vi "top_loop.vi"(0 "Input parameters":T4={"Measurement type"=enum."Debug", "Sensor type"=enum."HPK_8in_271ch", "Identifier"="test.txt", "Open after execution?"=FALSE, "Plot after execution?"=FALSE, "Display channel"=0, "Voltage Delay (s)"=0.5, "Switch Delay (s)"=0.01, "VISA resource name source"="", "VISA resource name DMM"="", "VISA resource name LCR"="", "Compliance  Level (A)"=10.0, "Voltage Limit (V)"=1000.0, "Data storage location"="", "Scan voltages"="", "Use source as DMM?"=FALSE, "LCR signal frequenzy (Hz)"=10.0, "DMM device"=enum."Keithley2001", "Sampling number"=1, "Use env. sensors on"=enum."Sensirion sht1x/7x", "Switchboard Handle"=0, "Use Switchboard"=FALSE, "LCR signal voltage (V)"=10000.0, "Repeat"=1, "Scan voltages IV"="", "Scan voltages CV"="", "Hex pad numbers?"=FALSE, "Set measurement type"=enum."Debug", "Custom pad scan"="", "IV voltage Delay (s)"=0.5, "CV voltage Delay (s)"=0.5, "Needle measurement?"=FALSE, "Comments"="test.txt", "LCR signal frequenzy (kHz)"=10.0, "Compliance  Level (uA)"=10.0, "Open Correction Array"=array2304x3[6912 elements], "Current set voltage"=0.0, "Last set voltage"=0.0, "Current channel"=0, "Last OpenCorrection index"=-1, "Total curr/vltg every x steps"=10, "Current channel iteration"=0, "No CV corrections"=FALSE, "Mapfile"="", "Corrfile"="", "IV voltage file"=path "", "CV voltage file"=path "", "IV Switch Delay (s)"=0.01, "CV Switch Delay (s)"=0.01, "Invert polarity"=FALSE, "Set debug dirs"=FALSE, "Is n on p"=FALSE, "Source interlock?"=TRUE, "Voltage file used?"=FALSE, "Pad mask"="", "Mask pad above (uA)"=1.0, "LCR device"=enum."LCR_E4980", "Source device"=enum."Source_2410", "HexPlot binary path"="", "PadReductionFactor"=1.0, "Temperature degC"="", "Fluence [neq]"="", "Annealing [min]"=""} {"CV Switch Delay (s)" format="%#_13g"; "IV Switch Delay (s)" format="%#_13g"; "Last set voltage" format="%#_13g"; "Current set voltage" format="%#_13g"; "CV voltage Delay (s)" format="%#_13g"; "IV voltage Delay (s)" format="%#_13g"; "Voltage Limit (V)" format="%#_13g"; "Voltage Delay (s)" format="%#_13g"; "Switch Delay (s)" format="%#_13g"}, 2 "?":refnum<k7>(container), 5 "Dynamic data":T3, 7 "Front_panel_refs":T2, 11 "error in (no error)":errorcluster, 12 "Environmental data":T1) -> (4 "Input parameters out":T4={"Measurement type"=enum."Debug", "Sensor type"=enum."HPK_8in_271ch", "Identifier"="test.txt", "Open after execution?"=FALSE, "Plot after execution?"=FALSE, "Display channel"=0, "Voltage Delay (s)"=0.5, "Switch Delay (s)"=0.01, "VISA resource name source"="", "VISA resource name DMM"="", "VISA resource name LCR"="", "Compliance  Level (A)"=10.0, "Voltage Limit (V)"=1000.0, "Data storage location"="", "Scan voltages"="", "Use source as DMM?"=FALSE, "LCR signal frequenzy (Hz)"=10.0, "DMM device"=enum."Keithley2001", "Sampling number"=1, "Use env. sensors on"=enum."Sensirion sht1x/7x", "Switchboard Handle"=0, "Use Switchboard"=FALSE, "LCR signal voltage (V)"=10000.0, "Repeat"=1, "Scan voltages IV"="", "Scan voltages CV"="", "Hex pad numbers?"=FALSE, "Set measurement type"=enum."Debug", "Custom pad scan"="", "IV voltage Delay (s)"=0.5, "CV voltage Delay (s)"=0.5, "Needle measurement?"=FALSE, "Comments"="test.txt", "LCR signal frequenzy (kHz)"=10.0, "Compliance  Level (uA)"=10.0, "Open Correction Array"=array2304x3[6912 elements], "Current set voltage"=0.0, "Last set voltage"=0.0, "Current channel"=0, "Last OpenCorrection index"=-1, "Total curr/vltg every x steps"=10, "Current channel iteration"=0, "No CV corrections"=FALSE, "Mapfile"="", "Corrfile"="", "IV voltage file"=path "", "CV voltage file"=path "", "IV Switch Delay (s)"=0.01, "CV Switch Delay (s)"=0.01, "Invert polarity"=FALSE, "Set debug dirs"=FALSE, "Is n on p"=FALSE, "Source interlock?"=TRUE, "Voltage file used?"=FALSE, "Pad mask"="", "Mask pad above (uA)"=1.0, "LCR device"=enum."LCR_E4980", "Source device"=enum."Source_2410", "HexPlot binary path"="", "PadReductionFactor"=1.0, "Temperature degC"="", "Fluence [neq]"="", "Annealing [min]"=""} {"CV Switch Delay (s)" format="%#_13g"; "IV Switch Delay (s)" format="%#_13g"; "Last set voltage" format="%#_13g"; "Current set voltage" format="%#_13g"; "CV voltage Delay (s)" format="%#_13g"; "IV voltage Delay (s)" format="%#_13g"; "Voltage Limit (V)" format="%#_13g"; "Voltage Delay (s)" format="%#_13g"; "Switch Delay (s)" format="%#_13g"}, 6 "Dynamic data out":T3, 8 "Front_panel_refs out":T2, 15 "error out":errorcluster)   [LabVIEW 2020]
doc: "The main loop function of the HexDAQ."
uses:
  input_params.ctl
  data_dynamic.ctl
  refs_front_panel.ctl
  <extravilib>/ChannelInstances/Tag-t'data_env.ctl'/))Channel.ctl
  data_env.ctl
  data_live.ctl
  <extravilib>/ChannelInstances/Tag-t'data_env.ctl'/Read With Abort.vi
  <extravilib>/ChannelInstances/Tag-t'data_env.ctl'/EndpointRead.vi
  <extravilib>/ChannelInstances/Tag-t'data_env.ctl'.lvlib
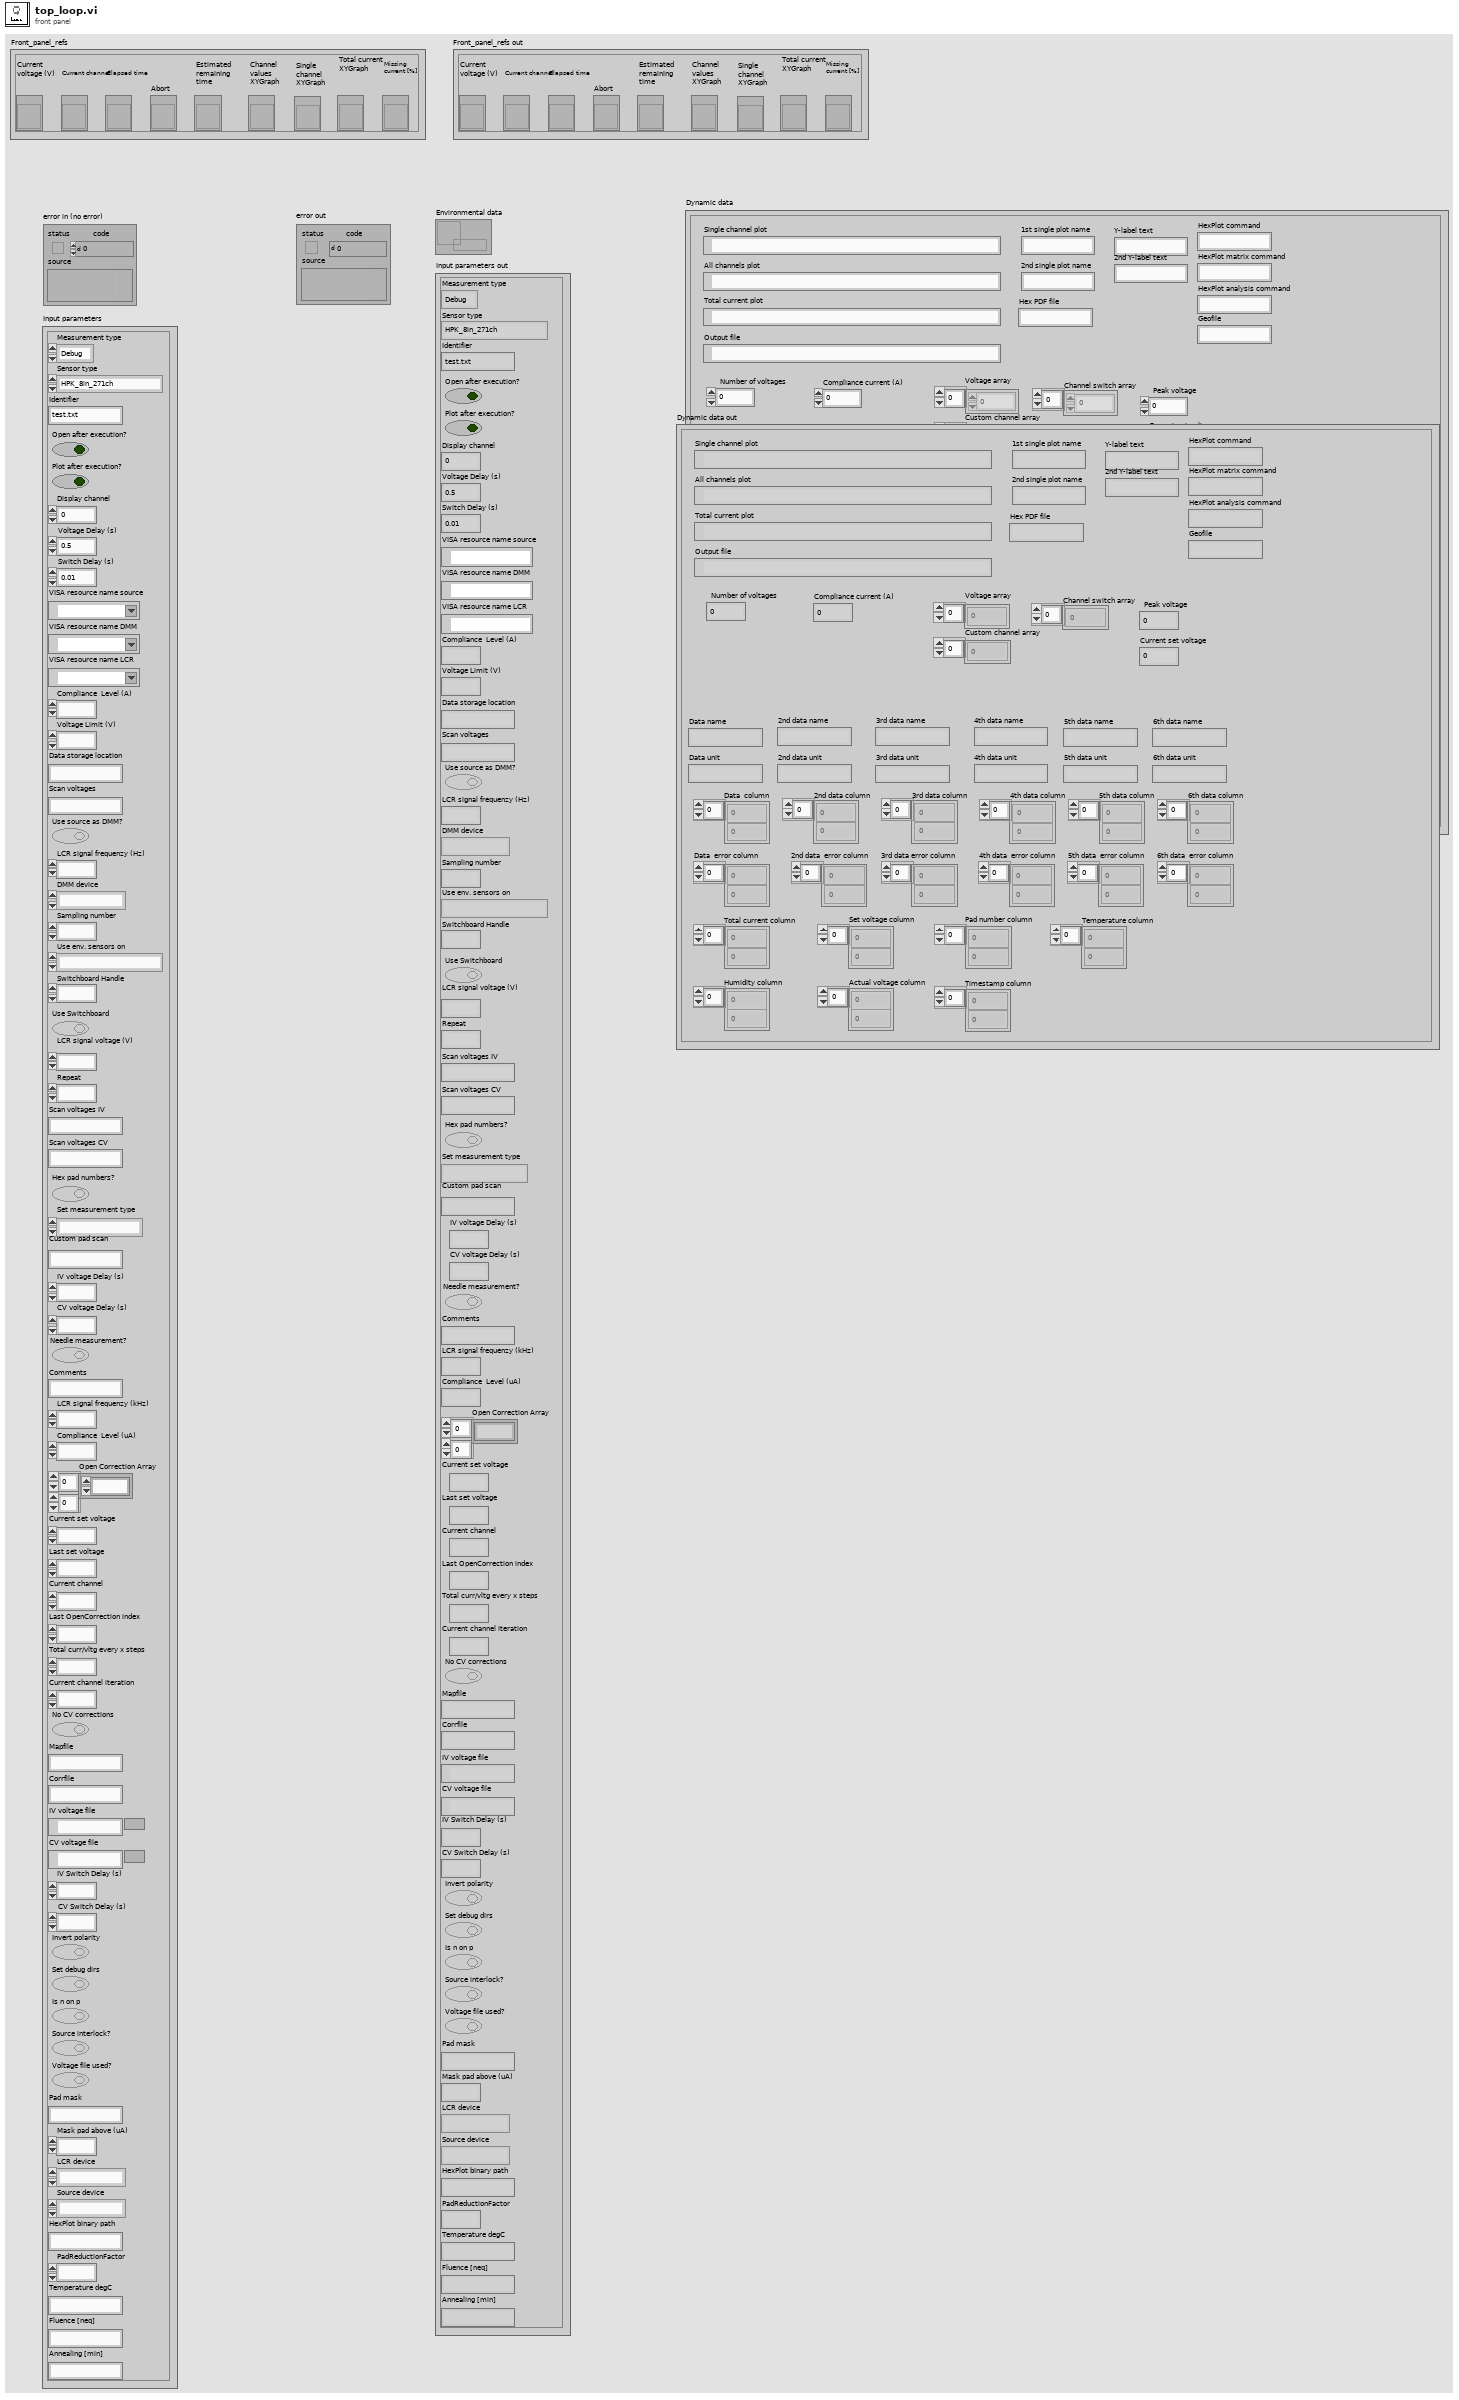
[diagram p1: front panel]
types:
  T1 = typedef "Tag-t'data_env.ctl'.lvlib/))Channel.ctl" = refnum<queue>
  T2 = typedef "refs_front_panel.ctl" = cluster{"Current voltage (V)":refnum<vi>, "Elapsed time":refnum<vi>, "Current channel":refnum<vi>, "Abort":refnum<vi>, "Estimated remaining time":refnum<vi>, "Channel values XYGraph":refnum<vi>, "Single channel XYGraph":refnum<vi>, "Total current XYGraph":refnum<vi>, "Missing\ncurrent [%]":refnum<vi>}
  T3 = typedef "data_dynamic.ctl" = cluster{"Output file":path, "Y-label text":string, "Current set voltage":dbl, "Set voltage column":dbl[], "Pad number column":dbl[], "Data  column":dbl[], "Number of voltages":i32, "Compliance current (A)":dbl, "Geofile":string, "Peak voltage":dbl, "Hex PDF file":string, "Voltage array":dbl[], "Total current column":dbl[], "Timestamp column":dbl[], "Data name":string, "Data unit":string, "2nd data column":dbl[], "2nd data name":string, "2nd data unit":string, "3rd data column":dbl[], "4th data column":dbl[], "3rd data name":string, "3rd data unit":string, "4th data name":string, "4th data unit":string, "Actual voltage column":dbl[], "2nd Y-label text":string, "Single channel plot":path, "Temperature column":dbl[], "Humidity column":dbl[], "Channel switch array":i32[], "1st single plot name":string, "2nd single plot name":string, "All channels plot":path, "HexPlot command":string, "Custom channel array":i32[], "Data  error column":dbl[], "2nd data  error column":dbl[], "3rd data error column":dbl[], "4th data  error column":dbl[], "Total current plot":path, "5th data column":dbl[], "5th data  error column":dbl[], "6th data column":dbl[], "6th data  error column":dbl[], "5th data name":string, "5th data unit":string, "6th data name":string, "6th data unit":string, "HexPlot matrix command":string, "HexPlot analysis command":string}
  T4 = typedef "input_params.ctl" = cluster{"Measurement type":enum16{"IV", "CV", "Debug", "Test_contact"}, "Sensor type":enum16{"HPK_6in_135ch", "HPK_8in_271ch", "IFX_8in_256ch", "Diode", "HPK_6in_239ch", "Full_Matrix", "HPK_8in_271ch_full", "LumiCal", "HPK_8in_444ch", "HPK_8in_198ch_2019", "HPK_8in_MGW_LD_full", "HPK_8in_MGW_LD_a_type_top", "HPK_8in_MGW_LD_a_type_bottom", "HPK_8in_MGW_LD_b_type_left", "HPK_8in_MGW_LD_b_type_right", "HPK_8in_MGW_LD_c_type_left", "HPK_8in_MGW_LD_c_type_right", "HPK_8in_MGW_HD_full", "HPK_8in_MGW_HD_a_type_top", "HPK_8in_MGW_HD_a_type_bottom", "HPK_8in_MGW_HD_b_type_left", "HPK_8in_MGW_HD_b_type_right", "HPK_8in_MGW_HD_c_type_left", "HPK_8in_MGW_HD_c_type_right", "CALICE_6in_256ch"}, "Identifier":string, "Open after execution?":bool, "Plot after execution?":bool, "Display channel":i32, "Voltage Delay (s)":dbl, "Switch Delay (s)":dbl, "VISA resource name source":refnum<visa-resource-name>, "VISA resource name DMM":refnum<visa-resource-name>, "VISA resource name LCR":refnum<visa-resource-name>, "Compliance  Level (A)":dbl, "Voltage Limit (V)":dbl, "Data storage location":string, "Scan voltages":string, "Use source as DMM?":bool, "LCR signal frequenzy (Hz)":dbl, "DMM device":enum16{"Keithley2001", "Keithley2450", "Keithley2410", "Keithley6485", "Keithley6487", "Keithley6517"}, "Sampling number":i32, "Use env. sensors on":enum16{"Sensirion sht1x/7x", "Switch Matrix", "Probecard"}, "Switchboard Handle":u32, "Use Switchboard":bool, "LCR signal voltage (V)":dbl, "Repeat":i32, "Scan voltages IV":string, "Scan voltages CV":string, "Hex pad numbers?":bool, "Set measurement type":enum16{"IV", "CV", "Debug", "Test_contact", "IV+CV"}, "Custom pad scan":string, "IV voltage Delay (s)":dbl, "CV voltage Delay (s)":dbl, "Needle measurement?":bool, "Comments":string, "LCR signal frequenzy (kHz)":dbl, "Compliance  Level (uA)":dbl, "Open Correction Array":dbl[][], "Current set voltage":dbl, "Last set voltage":dbl, "Current channel":i32, "Last OpenCorrection index":i32, "Total curr/vltg every x steps":i32, "Current channel iteration":i32, "No CV corrections":bool, "Mapfile":string, "Corrfile":string, "IV voltage file":path, "CV voltage file":path, "IV Switch Delay (s)":dbl, "CV Switch Delay (s)":dbl, "Invert polarity":bool, "Set debug dirs":bool, "Is n on p":bool, "Source interlock?":bool, "Voltage file used?":bool, "Pad mask":string, "Mask pad above (uA)":dbl, "LCR device":enum16{"LCR_E4980", "AGILENT_4263X"}, "Source device":enum16{"Source_2410", "Source_6487"}, "HexPlot binary path":string, "PadReductionFactor":dbl, "Temperature degC":string, "Fluence [neq]":string, "Annealing [min]":string}
  T5 = typedef "data_live.ctl" = cluster{"Actual voltage":dbl, "Total current":dbl, "Data":dbl, "Data error":dbl, "2nd data":dbl, "2nd data error":dbl, "3rd data":dbl, "3rd data error":dbl, "4th data":dbl, "4th data error":dbl, "6th data error":dbl, "6th data":dbl, "5th data error":dbl, "5th data":dbl}
  T6 = enum16{"Sensirion sht1x/7x", "Switch Matrix", "Probecard"}
  T7 = typedef "data_env.ctl" = cluster{"Temp. Sensirion":dbl, "Hum. Sensirion":dbl, "Temp. Switch Matrix":dbl, "Hum. Switch Matrix":dbl, "Temp. Probecard":dbl, "Hum. Probecard":dbl}
  T8 = cluster{"XY Graph out":cluster{"Array":dbl[], "Array":dbl[]}[], "XY Graph out":cluster{"Array":dbl[], "Array":dbl[]}[]}
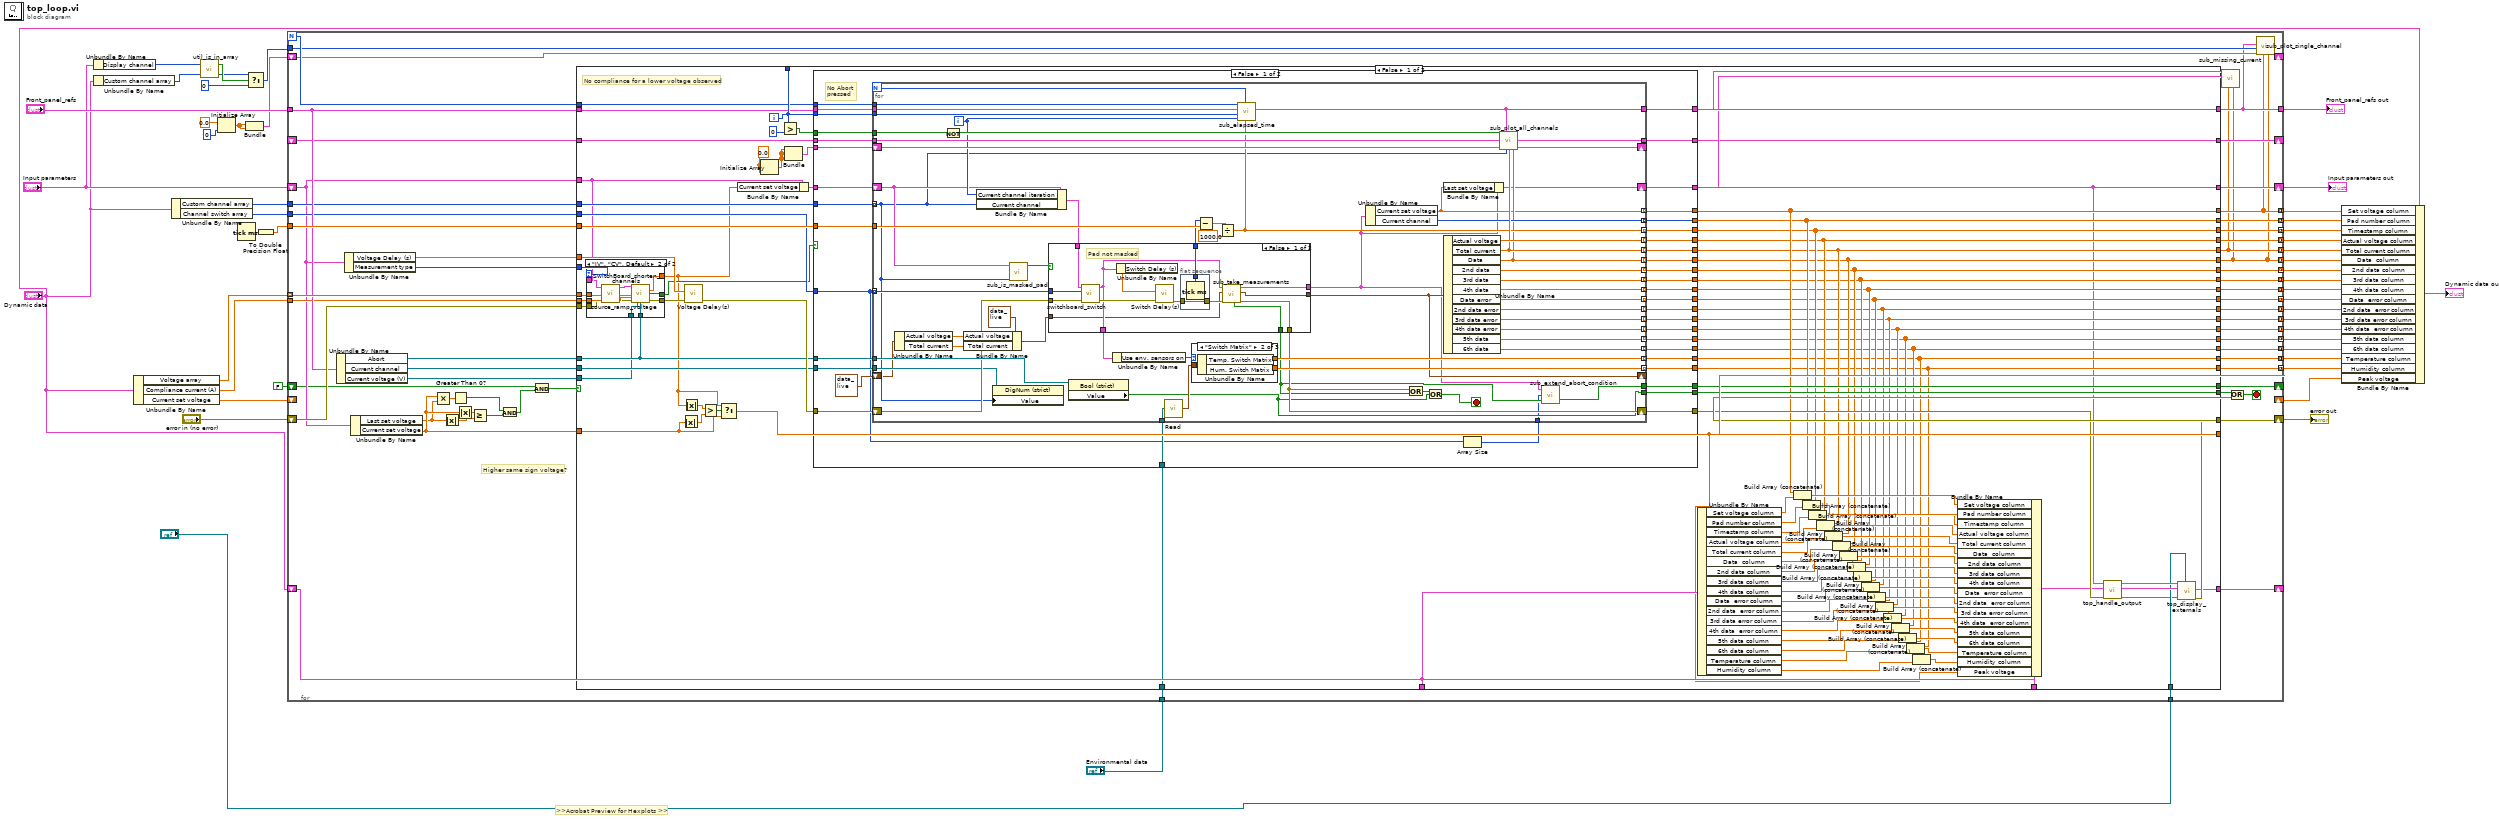
[diagram p0: block diagram]
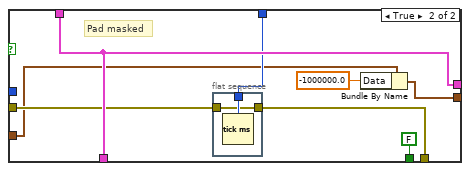
[diagram p2: hidden frame]
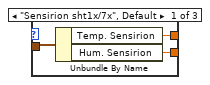
[diagram p3: hidden frame]
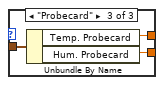
[diagram p4: hidden frame]
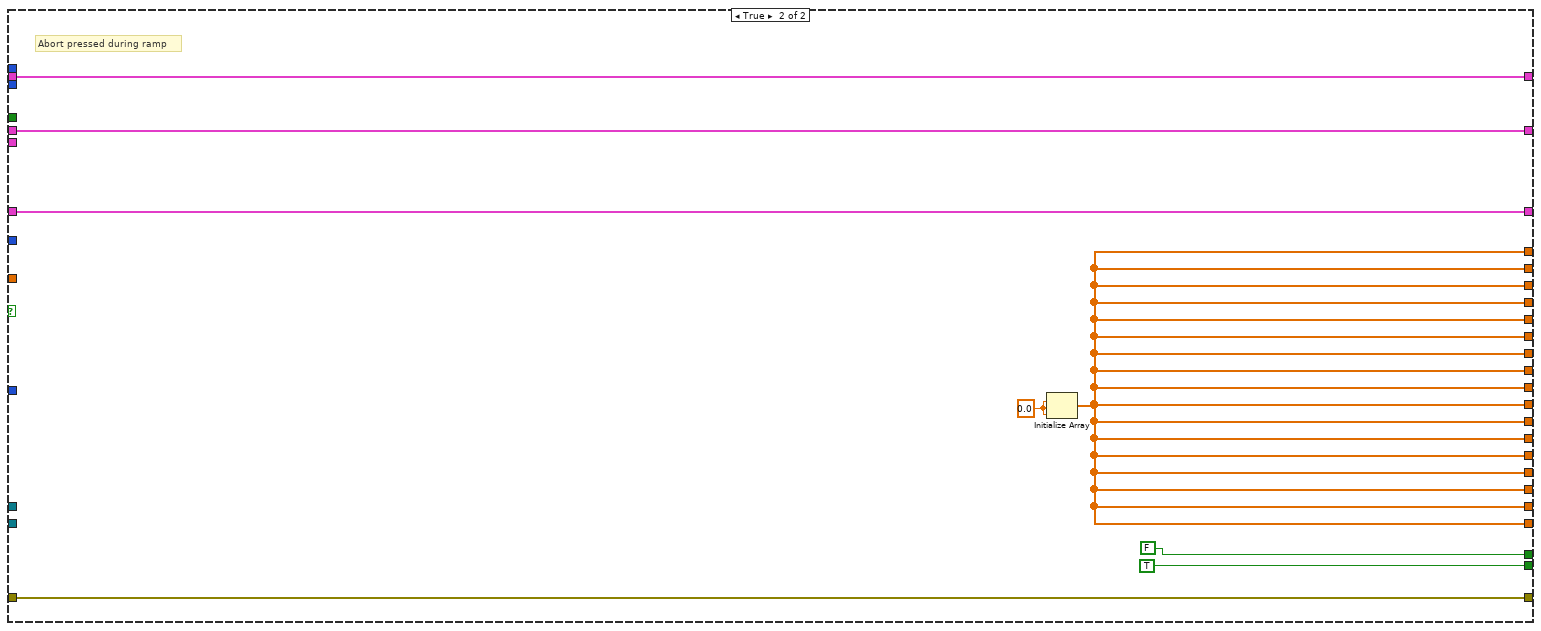
[diagram p5: hidden frame]
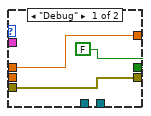
[diagram p6: hidden frame]
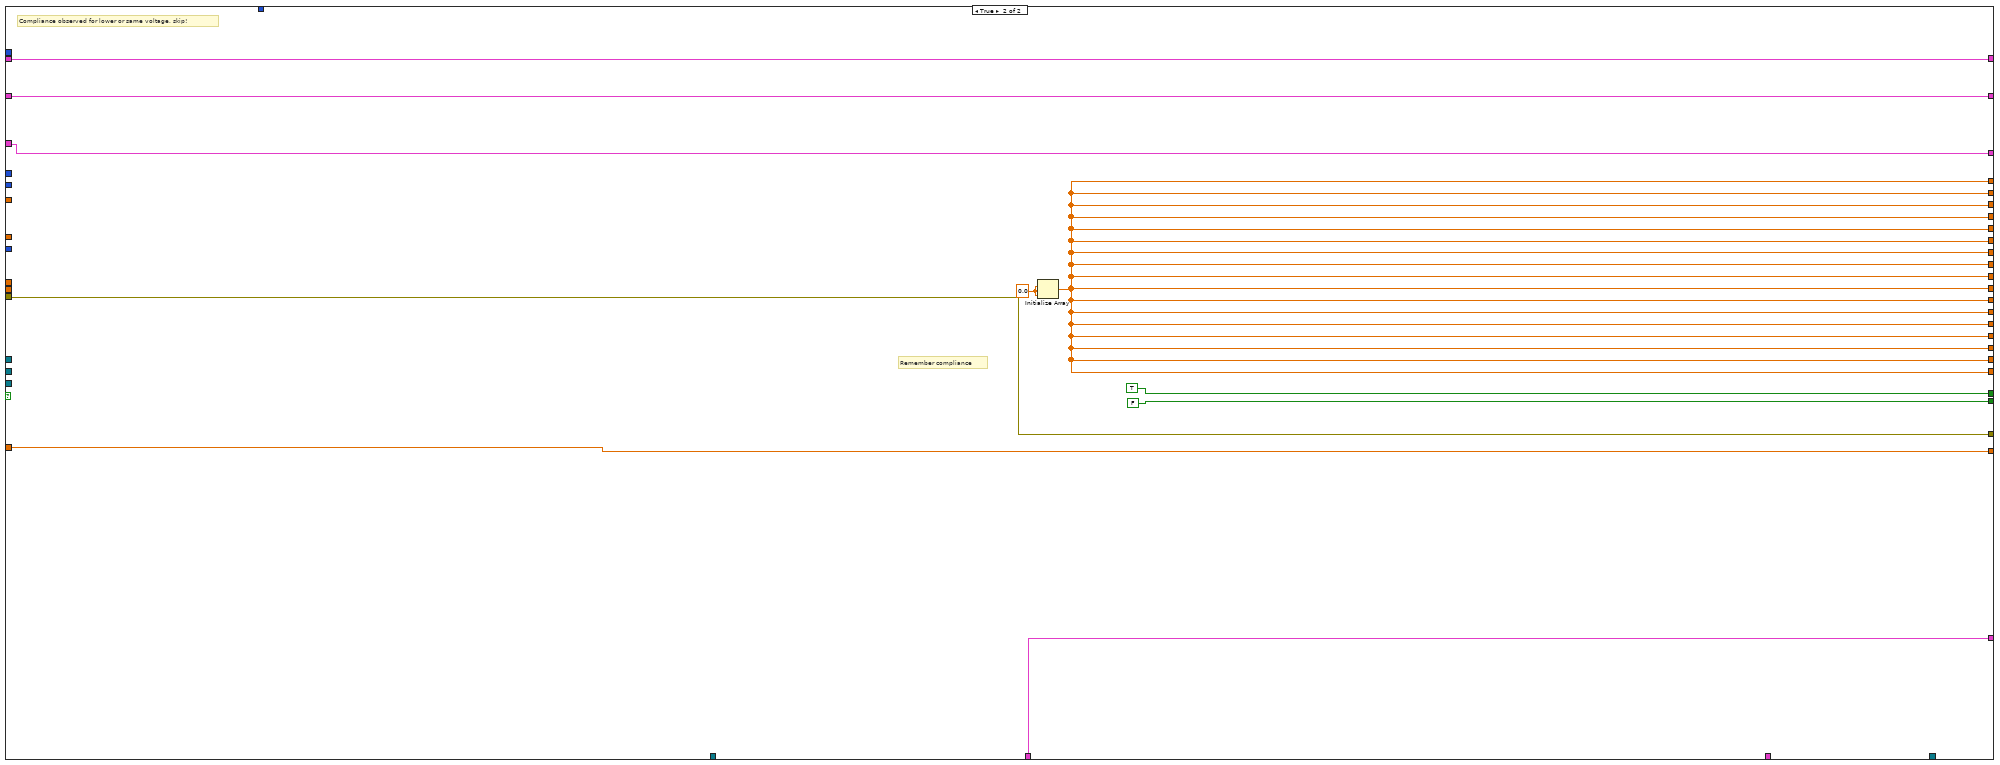
[diagram p7: hidden frame]
diagram:
  # ">>Acrobat Preview for Hexplots >>"
  n1 = Unbundle By Name("Input parameters") -> ("Display channel"=w25:i32)
  n2 = Unbundle By Name("Dynamic data") -> ("Custom channel array"=w24:i32[])
  n3 = Unbundle By Name("Dynamic data") -> ("Voltage array"=w26:dbl[], "Compliance current (A)"=w8:dbl, "Current set voltage"=w16:dbl)
  n4 = Unbundle By Name("Dynamic data") -> ("Custom channel array"=w21:i32[], "Channel switch array"=w20:i32[])
  n5 = call "util_is_in_array.vi"("Array"=w24, "Numeric"=w25) -> ("Position"=w5:i32, "Contains element?"=w6:bool)
  n6 = Initialize Array(0.0 ("Secondary Parameter"), 0 ("dimension size")) -> (w18:dbl[])
  n7 = Tick Count (ms)() -> (millisecond timer value=w28:u32)
  n8 = Bundle(w18, w18) -> (w17:cluster{dbl[], dbl[]})  [unwired: 1 in]
  n9 = Select(t=w5, s=w6, f=0 ("t")) -> (s? t:f=w22:i32)
  n10 = To Double Precision Float(number=w28) -> (double precision float=w27:dbl)
  n11 = for {
    N -> [w98]
    tunnel: w26 -> [w102] mode=indexing
    tunnel: [w67] -> w13 mode=concatenating
    tunnel: [w62] -> w46 mode=concatenating
    tunnel: [w66] -> w12 mode=concatenating
    shift-right: [w47] -> w43
    shift-left: "error in (no error)" -> [w104]
    shift-right: [w69] -> w44
    shift-left: "Input parameters" -> [w82]
    tunnel: w27 -> [w100]
    shift-right: [w68] -> w38
    shift-left: w16 -> [_]
    tunnel: [w63] -> w14 mode=concatenating
    tunnel: [w65] -> w15 mode=concatenating
    tunnel: [w61] -> w42 mode=concatenating
    tunnel: [w60] -> w41 mode=concatenating
    tunnel: [w59] -> w40 mode=concatenating
    tunnel: [w64] -> w39 mode=concatenating
    tunnel: [w52] -> w37 mode=concatenating
    tunnel: [w51] -> w36 mode=concatenating
    tunnel: "Environmental data" -> [w97]
    tunnel: [w58] -> w33 mode=concatenating
    tunnel: [w57] -> w32 mode=concatenating
    tunnel: [w56] -> w31 mode=concatenating
    tunnel: [w55] -> w30 mode=concatenating
    tunnel: "Front_panel_refs" -> [w95]
    tunnel: w22 -> [w84]
    tunnel: w8 -> [w91]
    tunnel: w21 -> [w90]
    tunnel: w20 -> [w89]
    shift-right: [w88] -> _
    shift-left: _ -> [w87]
    shift-right: [w85] -> _
    shift-left: w17 -> [w86]
    tunnel: [w53] -> w11 mode=concatenating
    tunnel: [w54] -> w10 mode=concatenating
    tunnel: [w78] -> w9
    shift-right: [w81] -> _
    shift-left: FALSE ("Value") -> [w80]
    tunnel: "?" -> [w49]
    shift-right: [w48] -> _
    shift-left: "Dynamic data" -> [w50]
    i -> [w99]
    stop <- w103 stop-if-true
    # "Higher same sign voltage?"
    n12 = Unbundle By Name(w95) -> ("Abort"=w96:refnum<vi>, "Current channel"=w93:refnum<vi>, "Current voltage (V)"=w94:refnum<vi>)
    n13 = Unbundle By Name(w82) -> ("Voltage Delay (s)"=w92:dbl, "Measurement type"=w101:enum16{"IV", "CV", "Debug", "Test_contact"})
    n14 = Unbundle By Name(w82) -> ("Last set voltage"=w73:dbl, "Current set voltage"=w74:dbl)
    n15 = Multiply(x=w74, y=w73) -> (x*y=w75:dbl)
    n16 = Absolute Value(x=w73) -> (abs(x)=w77:dbl)
    n17 = Greater Than 0?(x=w75) -> (x > 0?=w72:bool)
    n18 = Absolute Value(x=w74) -> (abs(x)=w76:dbl)
    n19 = Greater Or Equal?(x=w76, y=w77) -> (x >= y?=w71:bool)
    n20 = And(x=w72, y=w71) -> (x .and. y?=w70:bool)
    n21 = And(x=w80, y=w70) -> (x .and. y?=w79:bool)
    n22 = case shown="False" w79 {
      tunnel: [w124 w362] -> w66
      tunnel: w104 -> [w201 w366]
      tunnel: [w126 w367] -> w68
      tunnel: w102 -> [w198 _]
      tunnel: w101 -> [w197 _]
      tunnel: [w121 w362] -> w63
      tunnel: w100 -> [w195 _]
      tunnel: [w123 w362] -> w65
      tunnel: [w119 w362] -> w61
      tunnel: w99 -> [w194 _]
      tunnel: w98 -> [w193 _]
      tunnel: [w118 w362] -> w60
      tunnel: [w117 w362] -> w59
      tunnel: [w122 w362] -> w64
      tunnel: [w110 w362] -> w52
      tunnel: [w109 w362] -> w51
      tunnel: w97 -> [w192 _]
      tunnel: [w125 w362] -> w67
      tunnel: [w120 w362] -> w62
      tunnel: [w116 w362] -> w58
      tunnel: [w115 w362] -> w57
      tunnel: [w114 w362] -> w56
      tunnel: [w113 w362] -> w55
      tunnel: w96 -> [w190 _]
      tunnel: w95 -> [w189 w363]
      tunnel: [w107 w365] -> w69
      tunnel: w94 -> [w106 _]
      tunnel: w93 -> [w188 _]
      tunnel: w92 -> [w187 _]
      tunnel: w91 -> [w186 _]
      tunnel: w90 -> [w185 _]
      tunnel: w89 -> [w184 _]
      tunnel: [w181 w364] -> w88
      tunnel: w87 -> [w180 w364]
      tunnel: [w178 FALSE ("Value")] -> w83
      tunnel: [w162 w366] -> w47
      tunnel: [w111 w362] -> w53
      tunnel: [w112 w362] -> w54
      tunnel: w82 -> [w105 w365]
      tunnel: [w172 w363] -> w78
      tunnel: [w171 TRUE ("Value")] -> w81
      tunnel: w74 -> [w170 w367]
      tunnel: w50 -> [w169 w359]
      tunnel: w50 -> [w166 _]
      tunnel: w49 -> [w165 _]
      tunnel: [w108 w359] -> w48
      frame False {
        w191 = 0.0 ("dimension size")
        # "No compliance for a lower voltage observed"
        n23 = case shown="\"IV\", \"CV\", Default" w197 {
          tunnel: w198 -> [w346 w357]
          tunnel: w201 -> [w347 w352]
          tunnel: [w347 w358] -> w200
          tunnel: w186 -> [_ w356]
          tunnel: [w346 w355] -> w173
          tunnel: w190 -> [_ w353]
          tunnel: [FALSE ("Aborted?") w354] -> w177
          tunnel: w105 -> [_ w351]
          tunnel: w106 -> [_ w348]
          frame "Debug" {
          }
          frame "IV", "CV", Default {
            n24 = call "SwitchBoard_shorten_channels.vi"("error in"=w352, "Input parameters in"=w351) -> ("error out"=w349:errorcluster, "Input parameters out"=w350:T4)  [unwired: 8 in]
            n25 = call "source_ramp_voltage.vi"("Input parameters"=w350, "Target voltage (V)"=w357, "Compliance Current (A)"=w356, "error in (no error)"=w349, "Current source voltage reference"=w348, "Stop"=w353) -> ("Current voltage out (V)"=w355:dbl, "Aborted?"=w354:bool, "error out"=w358:errorcluster)  [unwired: 6 in, 1 out]
          }
        }
        n26 = Absolute Value(x=w170) -> (abs(x)=w174:dbl)
        n27 = Absolute Value(x=w173) -> (abs(x)=w175:dbl)
        n28 = call "Voltage Delay(s)"("error in (no error)"=w200, "Delay Time (s)"=w187) -> ("error out"=w196:errorcluster)  [unwired: 9 in]
        n29 = Greater?(x=w175, y=w174) -> (0:w176:bool)
        n30 = Select(t=w173, s=w176, f=w170) -> (s? t:f=w126:dbl)
        n31 = Bundle By Name(cluster=w105, "Current set voltage"=w173) -> (w179:T4)
        n32 = Initialize Array(w191, w191) -> (w183:dbl[])
        n33 = Greater?(x=w194, y=0) -> (0:w199:bool)
        n34 = Bundle(w183, w183, w183) -> (w182:cluster{dbl[], dbl[], dbl[]})  [unwired: 1 in]
        n35 = case shown="False" w177 {
          tunnel: [w241 w339] -> w124
          tunnel: w199 -> [w240 _]
          tunnel: w196 -> [w239 w342]
          tunnel: [w238 w339] -> w121
          tunnel: w195 -> [w237 _]
          tunnel: [w236 w339] -> w123
          tunnel: [w235 w339] -> w119
          tunnel: w194 -> [w234 _]
          tunnel: w193 -> [w233 _]
          tunnel: [w232 w339] -> w118
          tunnel: [w231 w339] -> w117
          tunnel: [w230 w339] -> w122
          tunnel: [w229 w339] -> w110
          tunnel: [w228 w339] -> w109
          tunnel: w192 -> [w227 _]
          tunnel: [w226 w339] -> w125
          tunnel: [w225 w339] -> w120
          tunnel: [w224 w339] -> w116
          tunnel: [w223 w339] -> w115
          tunnel: [w222 w339] -> w114
          tunnel: [w221 w339] -> w113
          tunnel: w190 -> [w220 _]
          tunnel: w189 -> [w219 w338]
          tunnel: [w218 w344] -> w107
          tunnel: w188 -> [w217 _]
          tunnel: w185 -> [w216 _]
          tunnel: w184 -> [w203 _]
          tunnel: w182 -> [w215 _]
          tunnel: [w214 w343] -> w181
          tunnel: w180 -> [w213 w343]
          tunnel: w179 -> [w212 w344]
          tunnel: [w211 TRUE ("Value")] -> w178
          tunnel: [w210 w342] -> w164
          tunnel: [w209 w339] -> w112
          tunnel: [w208 w339] -> w111
          tunnel: [w207 w338] -> w172
          tunnel: [w206 FALSE ("Value")] -> w171
          frame False {
            # "No Abort\npressed"
            n36 = Array Size(array=w203) -> (size(s)=w204:i32)
            n37 = for {
              N -> [w259]
              tunnel: w203 -> [w256] mode=indexing
              tunnel: [w271] -> w241 mode=indexing
              tunnel: [w269] -> w225 mode=indexing
              tunnel: [w262] -> w226 mode=indexing
              shift-right: [w268] -> w210
              shift-left: w239 -> [w292]
              tunnel: w240 -> [w286]
              tunnel: [w246] -> w211
              tunnel: w220 -> [w301]
              tunnel: [w275] -> w238 mode=indexing
              tunnel: w237 -> [w300]
              tunnel: [w273] -> w236 mode=indexing
              tunnel: [w285] -> w235 mode=indexing
              tunnel: w234 -> [w280]
              tunnel: w233 -> [w272]
              tunnel: [w297] -> w232 mode=indexing
              tunnel: [w296] -> w231 mode=indexing
              tunnel: [w295] -> w230 mode=indexing
              tunnel: [w294] -> w229 mode=indexing
              tunnel: [w293] -> w228 mode=indexing
              tunnel: w227 -> [w254]
              tunnel: w216 -> [w255] mode=indexing
              tunnel: [w290] -> w224 mode=indexing
              tunnel: [w289] -> w223 mode=indexing
              tunnel: [w288] -> w222 mode=indexing
              tunnel: [w287] -> w221 mode=indexing
              tunnel: w217 -> [w283]
              tunnel: w219 -> [w279]
              shift-right: [w278] -> _
              shift-left: w215 -> [w274]
              tunnel: [w276] -> w214
              tunnel: w213 -> [w277]
              shift-right: [w263] -> w218
              shift-left: w212 -> [w258]
              tunnel: [w265] -> w209 mode=indexing
              tunnel: [w264] -> w208 mode=indexing
              tunnel: [w260] -> w207
              tunnel: [w245] -> w206
              shift-right: [w252] -> _
              shift-left: T5 {"Actual voltage"=0.0, "Total current"=0.0, "Data"=0.0, "Data error"=0.0, "2nd data"=0.0, "2nd data error"=0.0, "3rd data"=0.0, "3rd data error"=0.0, "4th data"=0.0, "4th data error"=0.0, "6th data error"=0.0, "6th data"=0.0, "5th data error"=0.0, "5th data"=0.0} ("Live data out") -> [w251]
              tunnel: w204 -> [w242]
              i -> [w261]
              stop <- w266 stop-if-true
              n38 = Unbundle By Name(w251) -> ("Actual voltage"=w250:dbl, "Total current"=w247:dbl)
              n39 = Not(x=w286) -> (.not. x?=w284:bool)
              n40 = Bundle By Name(cluster=T5 {"Actual voltage"=0.0, "Total current"=0.0, "Data"=0.0, "Data error"=0.0, "2nd data"=0.0, "2nd data error"=0.0, "3rd data"=0.0, "3rd data error"=0.0, "4th data"=0.0, "4th data error"=0.0, "6th data error"=0.0, "6th data"=0.0, "5th data error"=0.0, "5th data"=0.0} ("Live data out"), "Actual voltage"=w250, "Total current"=w247) -> (w248:T5)
              n41 = Bundle By Name(cluster=w258, "Current channel iteration"=w261, "Current channel"=w255) -> (w270:T4)
              n42 = property on="Property Node" class="DigNum (strict)"(reference=w283, "Value"=w255) -> ()  [unwired: 1 in, 2 out]
              n43 = call "sub_is_masked_pad.vi"("Pad number"=w255, "Input parameters"=w258) -> ("Is masked?"=w257:bool)  [unwired: 9 in]
              n44 = case shown="False" w257 {
                tunnel: [w315 w323] -> w298
                tunnel: w292 -> [w312 w322]
                tunnel: w256 -> [w310 _]
                tunnel: [w308 w325] -> w281
                tunnel: w270 -> [w307 w325]
                tunnel: [w306 w321] -> w268
                tunnel: [w305 w325] -> w243
                tunnel: [w304 w318] -> w252
                tunnel: w248 -> [w303 w319]
                tunnel: [w302 FALSE ("Compliance reached?")] -> w244
                frame False {
                  # "Pad not masked"
                  n45 = call "switchboard_switch.vi"("error in"=w312, "Channel"=w310, "Input parameters in"=w307) -> ("error out"=w311:errorcluster, "Input parameters out"=w308:T4)  [unwired: 7 in]
                  n46 = Unbundle By Name(w308) -> ("Switch Delay (s)"=w309:dbl)
                  n47 = call "Switch Delay(s)"("error in (no error)"=w311, "Delay Time (s)"=w309) -> ("error out"=w314:errorcluster)  [unwired: 9 in]
                  n48 = flat-sequence {
                    tunnel: [w317] -> w315
                    tunnel: w314 -> [w316]
                    tunnel: [w316] -> w313
                    frame #0 {
                      n49 = Tick Count (ms)() -> (millisecond timer value=w317:u32)
                    }
                  }
                  n50 = call "sub_take_measurements.vi"("error in (no error)"=w313, "Live data in"=w303, "Input parameters"=w308) -> ("error out"=w306:errorcluster, "Live data out"=w304:T5, "Input parameters out"=w305:T4, "Compliance reached?"=w302:bool)  [unwired: 5 in]
                }
                frame True {
                  # "Pad masked"
                  n51 = flat-sequence {
                    tunnel: [w327] -> w323
                    tunnel: w322 -> [w326]
                    tunnel: [w326] -> w321
                    frame #0 {
                      n52 = Tick Count (ms)() -> (millisecond timer value=w327:u32)
                    }
                  }
                  n53 = Bundle By Name(cluster=w319, "Data"=-1000000.0 ("y")) -> (w318:T5)
                }
              }
              n54 = property class="Bool (strict)"(reference=w301) -> ("Value"=w246:bool)  [unwired: 1 in, 2 out]
              n55 = Unbundle By Name(w281) -> ("Use env. sensors on"=w291:T6)
              n56 = call <extravilib>:"Read.vi"("channel"=w254) -> ("element"=w253:T7)  [unwired: 1 in, 1 out]
              n57 = case shown="\"Switch Matrix\"" w291 {
                tunnel: w253 -> [w330 w333 w336]
                tunnel: [w329 w331 w334] -> w294
                tunnel: [w328 w332 w335] -> w293
                frame "Sensirion sht1x/7x", Default {
                  n58 = Unbundle By Name(w330) -> ("Temp. Sensirion"=w329:dbl, "Hum. Sensirion"=w328:dbl)
                }
                frame "Switch Matrix" {
                  n59 = Unbundle By Name(w333) -> ("Temp. Switch Matrix"=w331:dbl, "Hum. Switch Matrix"=w332:dbl)
                }
                frame "Probecard" {
                  n60 = Unbundle By Name(w336) -> ("Temp. Probecard"=w334:dbl, "Hum. Probecard"=w335:dbl)
                }
              }
              n61 = Subtract(x=w298, y=w300) -> (x-y=w282:dbl)
              n62 = Divide(x=w282, y=1000.0) -> (x/y=w273:dbl)
              n63 = call "sub_elapsed_time.vi"("Elapsed time (s)"=w273, "Inner N"=w259, "Inner i"=w261, "Outer i"=w280, "Front_panel_refs"=w279, "Outer N"=w272) -> ("Front_panel_refs out"=w260:T2)  [unwired: 5 in]
              n64 = Unbundle By Name(w243) -> ("Current set voltage"=w262:dbl, "Current channel"=w271:i32)
              n65 = Or(x=w268, y=w244) -> (x .or. y?=w267:bool)
              n66 = Or(x=w267, y=w246) -> (x .or. y?=w266:bool)
              n67 = Bundle By Name(cluster=w243, "Last set voltage"=w262) -> (w263:T4)
              n68 = Unbundle By Name(w252) -> ("Actual voltage"=w295:dbl, "Total current"=w275:dbl, "Data"=w269:dbl, "2nd data"=w285:dbl, "3rd data"=w297:dbl, "4th data"=w296:dbl, "Data error"=w290:dbl, "2nd data error"=w289:dbl, "3rd data error"=w288:dbl, "4th data error"=w287:dbl, "5th data"=w265:dbl, "6th data"=w264:dbl)
              n69 = call "sub_plot_all_channels.vi"("Is first?"=w284, "Front_panel_refs"=w260, "Plot cluster"=w277, "Cluster"=w274, "Custom channel"=w255, "Total current"=w275, "Data"=w269) -> ("Plot cluster out"=w276:T8, "Cluster out"=w278:cluster{dbl[], dbl[], dbl[]})  [unwired: 7 in]
              n70 = call "sub_extend_abort_condition.vi"("Abort(in)"=w244, "NTestChannels"=w242, "Input parameters"=w243) -> ("Abort(out)"=w245:bool)  [unwired: 1 out]
            }
          }
          frame True {
            w340 = 0.0 ("dimension size")
            # "Abort pressed during ramp"
            n71 = Initialize Array(w340, w340) -> (w339:dbl[])
          }
        }
        n72 = Unbundle By Name(w169) -> ("Set voltage column"=w160:dbl[], "Pad number column"=w159:dbl[], "Timestamp column"=w158:dbl[], "Actual voltage column"=w157:dbl[], "Total current column"=w156:dbl[], "Data  column"=w155:dbl[], "2nd data column"=w154:dbl[], "3rd data column"=w153:dbl[], "4th data column"=w152:dbl[], "Data  error column"=w151:dbl[], "2nd data  error column"=w150:dbl[], "3rd data error column"=w149:dbl[], "4th data  error column"=w148:dbl[], "5th data column"=w147:dbl[], "6th data column"=w146:dbl[], "Temperature column"=w145:dbl[], "Humidity column"=w144:dbl[])
        n73 = Build Array (concatenate)(w125, w160) -> (w143:dbl[])
        n74 = Build Array (concatenate)(w124, w159) -> (w142:dbl[])
        n75 = Build Array (concatenate)(w123, w158) -> (w141:dbl[])
        n76 = Build Array (concatenate)(w122, w157) -> (w140:dbl[])
        n77 = Build Array (concatenate)(w121, w156) -> (w139:dbl[])
        n78 = Build Array (concatenate)(w120, w155) -> (w138:dbl[])
        n79 = Build Array (concatenate)(w119, w154) -> (w137:dbl[])
        n80 = Build Array (concatenate)(w118, w153) -> (w136:dbl[])
        n81 = Build Array (concatenate)(w117, w152) -> (w135:dbl[])
        n82 = Build Array (concatenate)(w116, w151) -> (w134:dbl[])
        n83 = Build Array (concatenate)(w115, w150) -> (w133:dbl[])
        n84 = Build Array (concatenate)(w114, w149) -> (w132:dbl[])
        n85 = Build Array (concatenate)(w113, w148) -> (w131:dbl[])
        n86 = Build Array (concatenate)(w112, w147) -> (w130:dbl[])
        n87 = Build Array (concatenate)(w111, w146) -> (w129:dbl[])
        n88 = Build Array (concatenate)(w110, w145) -> (w128:dbl[])
        n89 = Build Array (concatenate)(w109, w144) -> (w127:dbl[])
        n90 = Bundle By Name(cluster=w166, "Set voltage column"=w143, "Pad number column"=w142, "Timestamp column"=w141, "Actual voltage column"=w140, "Total current column"=w139, "Data  column"=w138, "2nd data column"=w137, "3rd data column"=w136, "4th data column"=w135, "Data  error column"=w134, "2nd data  error column"=w133, "3rd data error column"=w132, "4th data  error column"=w131, "5th data column"=w130, "6th data column"=w129, "Temperature column"=w128, "Humidity column"=w127, "Peak voltage"=w126) -> (w161:T3)
        n91 = call "top_handle_output.vi"("error in (no error)"=w164, "Dynamic data"=w161, "Input parameters"=w107) -> ("error out"=w163:errorcluster, "Dynamic data"=w167:T3, "Input parameters"=w168:T4)  [unwired: 6 in]
        n92 = call "top_display_externals.vi"("AcroPDF"=w165, "error in (no error)"=w163, "Dynamic data"=w167, "Input parameters"=w168) -> ("error out"=w162:errorcluster, "Dynamic data"=w108:T3)  [unwired: 5 in, 1 out]
      }
      frame True {
        w368 = 0.0 ("dimension size")
        # "Remember compliance"
        # "Compliance observed for lower or same voltage, skip!"
        n93 = Initialize Array(w368, w368) -> (w362:dbl[])
      }
    }
    n94 = call "sub_missing_current.vi"("Data"=w62, "Total current"=w63, "Input parameters out"=w69, "Front_panel_refs"=w78) -> ()  [unwired: 8 in]
    n95 = Or(x=w83, y=w47) -> (x .or. y?=w103:bool)
    n96 = call "sub_plot_single_channel.vi"("Data column"=w62, "Set voltage column"=w67, "Cluster"=w86, "Channel"=w84, "Front_panel_refs"=w78) -> ("Cluster out"=w85:cluster{dbl[], dbl[]})  [unwired: 6 in]
  }
  "error out" <- w43
  "Input parameters out" <- w44
  "Front_panel_refs out" <- w9
  n97 = Bundle By Name(cluster="Dynamic data", "Set voltage column"=w13, "Pad number column"=w12, "Timestamp column"=w15, "Actual voltage column"=w39, "Total current column"=w14, "Data  column"=w46, "2nd data column"=w42, "3rd data column"=w41, "4th data column"=w40, "Data  error column"=w33, "2nd data  error column"=w32, "3rd data error column"=w31, "4th data  error column"=w30, "5th data column"=w10, "6th data column"=w11, "Temperature column"=w37, "Humidity column"=w36, "Peak voltage"=w38) -> (→"Dynamic data out":T3)
